vi "variantData.vi"() -> ()   [LabVIEW 2014]
panel:
  out "Raw (\"Flattened\")\nVariant Data":string
  out "Variant Type\nMetadata":i16[](array[numeric])
  out "Data Unpacked \nFrom Variant":i32
  out "Variant Atrribute\nValue":variant
  out "Found Requested\nVariant Attribute":bool
  out "Variant Operations\nError State":errorcluster
  out "Data Before Packing \nInto Variant":dbl=3.141592653589793
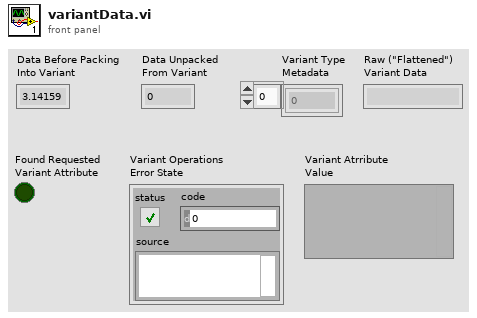
[diagram p1: front panel]
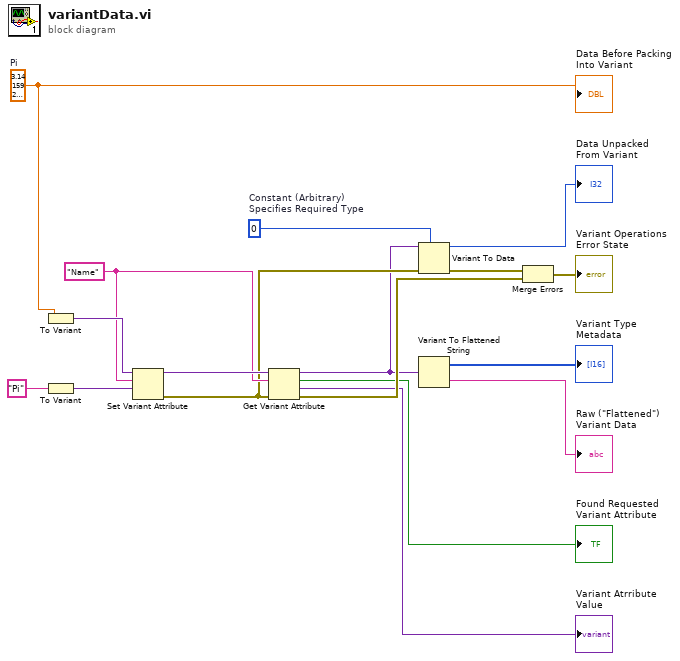
[diagram p0: block diagram]
diagram:
  w11 = "Name" ("name")
  w15 = 0  # Constant (Arbitrary) Specifies Required Type
  w17 = 3.141592653589793  # Pi
  n1 = To Variant(anything=w17) -> (Variant=w16:variant)
  n2 = To Variant(anything="Pi") -> (Variant=w13:variant)
  n3 = Set Variant Attribute(Variant=w16, name=w11, value=w13) -> (Variant out=w12:variant, error out=w10:errorcluster)  [unwired: 1 in, 1 out]
  n4 = Get Variant Attribute(Variant=w12, name=w11, error in=w10) -> (duplicate Variant=w3:variant, found=→"Found Requested\nVariant Attribute":bool, value=→"Variant Atrribute\nValue":variant, error out=w8:errorcluster)  [unwired: 1 in]
  n5 = Variant To Data(error in=w10, type=w15, Variant=w3) -> (data=→"Data Unpacked \nFrom Variant":i32, error out=w9:errorcluster)
  n6 = Variant To Flattened String(Variant=w3) -> (data string=→"Raw (\"Flattened\")\nVariant Data":string, 1:→"Variant Type\nMetadata":i16[])
  n7 = Merge Errors(w9, w8) -> (→"Variant Operations\nError State":errorcluster)
  "Data Before Packing \nInto Variant" <- w17
